vi "配置文件保存.vi"   [LabVIEW 2016, in "挥发酚.lvlib"]
uses:
  <vilib>/Utility/config.llb/NI_LVConfig.lvlib
types:
  T1 = typedef "NI_LVConfig.lvlib/Config Data RefNum.ctl" = refnum<k1>
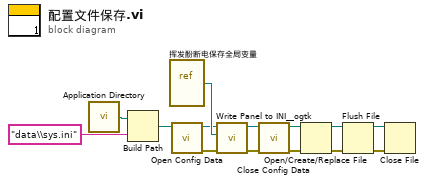
[diagram p0: block diagram]
diagram:
  n1 = call <vilib>:"Application Directory.vi"() -> ("Application Directory"=w2:path)
  n2 = Build Path(base path=w2, name or relative path="data\\sys.ini" ("名称或相对路径")) -> (appended path=w3:path)
  n3 = vi-ref "挥发酚断电保存全局变量.vi"() -> (w5:refnum<vi>)
  n4 = call <vilib>:"Open Config Data.vi"("configuration file path"=w3) -> ("error out"=w7:errorcluster, "refnum"=w4:T1)  [unwired: 8 in, 1 out]
  n5 = call <userlib>:"Write Panel to INI__ogtk.vi"("error in (no error)"=w7, "VI ref"=w5, "refnum"=w4) -> ("error out"=w8:errorcluster, "refnum out"=w6:T1)  [unwired: 7 in]
  n6 = call <vilib>:"Close Config Data.vi"("error in (no error)"=w8, "refnum"=w6) -> ("error out"=w13:errorcluster, "file path"=w14:path)  [unwired: 8 in]
  n7 = Open/Create/Replace File(file path (use dialog)=w14, error in=w13) -> (refnum out=w10:refnum<file>, error out=w9:errorcluster)  [unwired: 4 in, 1 out]
  n8 = Flush File(refnum=w10, error in=w9) -> (refnum out=w11:refnum<file>, error out=w12:errorcluster)
  n9 = Close File(refnum=w11, error in=w12) -> ()  [unwired: 2 out]
